vi "Load Grey Selector.vi"(8 "error in (no error)":errorcluster, 11 "ColorSelector in":refnum<class "ColorSelector.lvclass">) -> (0 "error out":errorcluster, 3 "ColorSelector out":refnum<class "ColorSelector.lvclass">)   [LabVIEW 2015, in "ColorSelector.lvclass"]
doc: "This VI draws the Grey Selector.\n<b> </b> <b> </b>\n©2017 Q Software Innovations, LLC (QSI)\nwritten by Quentin Alldredge\nproduced in LabVIEW 2015\n\nsupport@qsoftwareinnovations.com\nwww.qsoftwareinnovations.com\n\nAll rights reserved.\n\nRedistribution and use in source and binary forms, with or without modification, are permitted provided that the following conditions are met:\n\n * Redistributions of source code must retain the above copyright notice, this list of conditions and the following disclaimer.\n * Redistributions in binary form must reproduce the above copyright notice, this list of conditions and the following disclaimer in the documentation and/or other materials provided with the distribution.\n * Neither the name of Q Software Innovations, LLC. nor the names of its contributors may be used to endorse or promote products derived from this software without specific prior written permission.\n\nTHIS SOFTWARE IS PROVIDED BY THE COPYRIGHT HOLDERS AND CONTRIBUTORS \"AS IS\" AND ANY EXPRESS OR IMPLIED WARRANTIES, INCLUDING, BUT NOT LIMITED TO, THE IMPLIED WARRANTIES OF MERCHANTABILITY AND FITNESS FOR A PARTICULAR PURPOSE ARE DISCLAIMED. IN NO EVENT SHALL THE COPYRIGHT OWNER OR CONTRIBUTORS BE LIABLE FOR ANY DIRECT, INDIRECT, INCIDENTAL, SPECIAL, EXEMPLARY, OR CONSEQUENTIAL DAMAGES (INCLUDING, BUT NOT LIMITED TO, PROCUREMENT OF SUBSTITUTE GOODS OR SERVICES; LOSS OF USE, DATA, OR PROFITS; OR BUSINESS INTERRUPTION) HOWEVER CAUSED AND ON ANY THEORY OF LIABILITY, WHETHER IN CONTRACT, STRICT LIABILITY, OR TORT (INCLUDING NEGLIGENCE OR OTHERWISE) ARISING IN ANY WAY OUT OF THE USE OF THIS SOFTWARE, EVEN IF ADVISED OF THE POSSIBILITY OF SUCH DAMAGE."
uses:
  ColorSelector.lvclass
  <vilib>/picture/picture.llb/imagedata.ctl
  ColorSelector.lvclass/ColorSelector.ctl
  Write GreySelectPic.vi
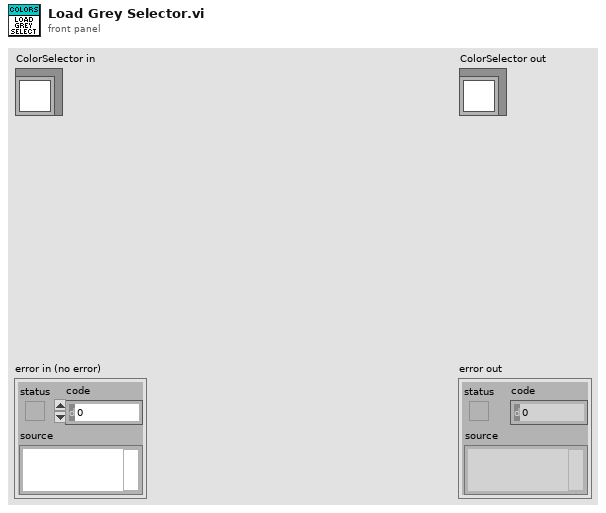
[diagram p1: front panel]
types:
  T1 = typedef "imagedata.ctl" = cluster{"image type":i32, "image depth":i32, "image":u8[], "mask":u8[], "colors":u32[], "Rectangle":cluster{"left":i16, "top":i16, "right":i16, "bottom":i16}}
  T2 = typedef "LVBoundsTypeDef.ctl" = cluster{"Width":u32, "Height":u32}
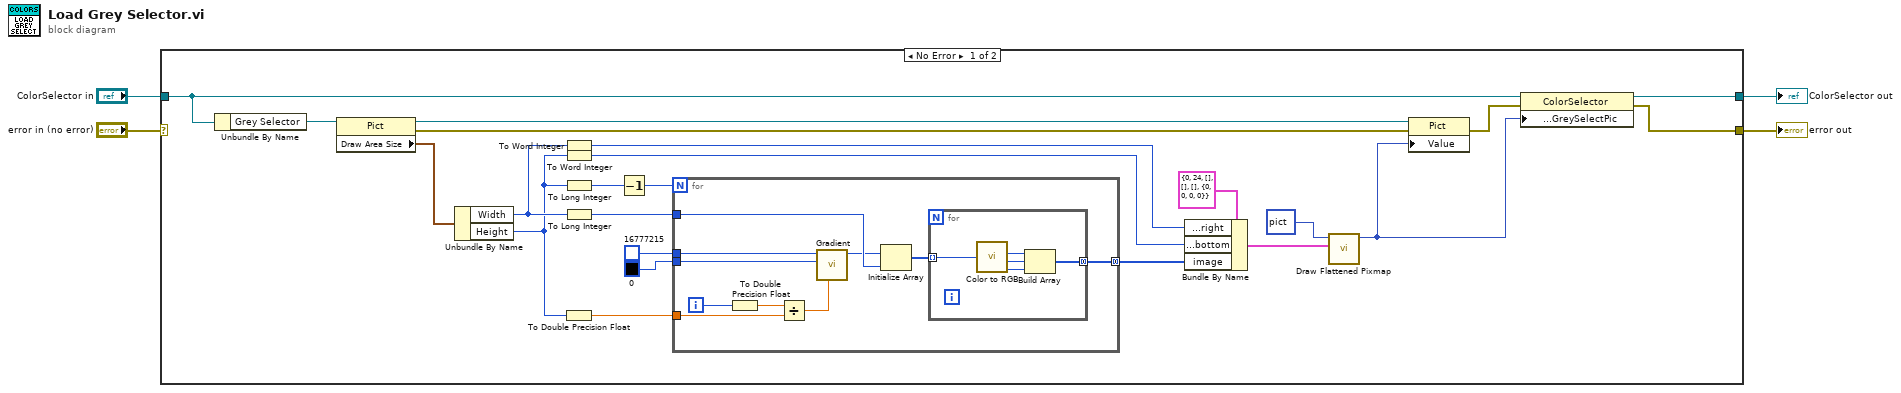
[diagram p0: block diagram]
diagram:
  n1 = case shown="No Error" "error in (no error)" {
    selector: "error in (no error)" -> [_ w44]
    tunnel: [w12 w44] -> w3
    tunnel: [w14 w43] -> w1
    tunnel: "ColorSelector in" -> [w27 w43]
    frame No Error {
      n2 = Unbundle By Name(w27) -> ("Grey Selector"=w26:refnum<vi>)
      n3 = property class="Pict"(reference=w26) -> (reference out=w25:refnum<vi>, error out=w24:errorcluster, "Draw Area Size"=w23:T2)  [unwired: 1 in]
      n4 = Unbundle By Name(w23) -> ("Width"=w18:u32, "Height"=w5:u32)
      n5 = To Word Integer(number=w18) -> (16bit integer=w16:i16)
      n6 = To Word Integer(number=w5) -> (16bit integer=w15:i16)
      n7 = To Long Integer(number=w5) -> (32bit integer=w6:i32)
      n8 = To Long Integer(number=w18) -> (32bit integer=w17:i32)
      n9 = To Double Precision Float(number=w5) -> (double precision float=w8:dbl)
      n10 = Decrement(x=w6) -> (x-1=w7:i32)
      n11 = for {
        N: w7 -> [_]
        tunnel: [w37] -> w22 mode=concatenating
        tunnel: w17 -> [w36]
        tunnel: u32 16777215 -> [w34]
        tunnel: u32 0 -> [w33]
        tunnel: w8 -> [w30]
        i -> [w32]
        n12 = To Double Precision Float(number=w32) -> (double precision float=w31:dbl)
        n13 = Divide(x=w31, y=w30) -> (x/y=w29:dbl)
        n14 = call "Gradient.vi"("Percent"=w29, "End Color"=w33, "Start Color"=w34) -> ("Gradient Color"=w28:u32)  [unwired: 8 in]
        n15 = Initialize Array(w28, w36) -> (w35:u32[])
        n16 = for {
          tunnel: [w39] -> w37 mode=concatenating
          tunnel: w35 -> [w38] mode=indexing
          n17 = call <vilib>:"Color to RGB.vi"("Color"=w38) -> ("R"=w42:u8, "G"=w41:u8, "B"=w40:u8)  [unwired: 1 out]
          n18 = Build Array(w42, w41, w40) -> (w39:u8[])
        }
      }
      n19 = Bundle By Name(cluster=T1 {"image type"=0, "image depth"=24, "image"=[], "mask"=[], "colors"=[], "Rectangle"={"left"=0, "top"=0, "right"=0, "bottom"=0}} ("image data"), "Rectangle.right"=w16, "Rectangle.bottom"=w15, "image"=w22) -> (w19:T1)
      n20 = call <vilib>:"Draw Flattened Pixmap.vi"("image data"=w19, "picture"=picture data[5B] ("new picture")) -> ("new picture"=w11:picture)  [unwired: 7 in]
      n21 = property class="Pict"(reference=w25, error in=w24, "Value"=w11) -> (error out=w13:errorcluster)  [unwired: 1 out]
      n22 = property class="ColorSelector"(reference=w27, error in=w13, "State Data:Accessors:GreySelectPic"=w11) -> (reference out=w14:refnum<class "ColorSelector.lvclass">, error out=w12:errorcluster)
    }
    frame Error {
    }
  }
  "error out" <- w3
  "ColorSelector out" <- w1
